vi "get runtime class name.vi"(8 "error in":errorcluster, 11 "configuration in":refnum<class "action configuration.lvclass">) -> (0 "error out":errorcluster, 2 "class name":string, 3 "configuration out":refnum<class "action configuration.lvclass">)   [LabVIEW 2014, in "action configuration.lvclass"]
doc: "Provides an interface for determining the runtime class associated with this configuration. This class name can then be used to dynamically load or locate the runtime class for initialization purposes."
uses:
  action configuration.lvclass
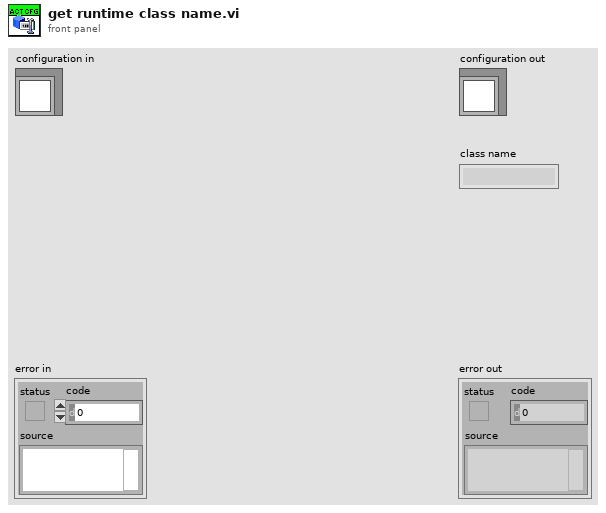
[diagram p1: front panel]
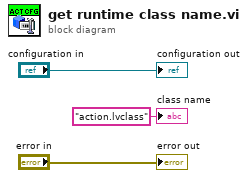
[diagram p0: block diagram]
diagram:
  "error out" <- "error in"
  "configuration out" <- "configuration in"
  "class name" <- "action.lvclass" ("class name")
